vi "Main.vi"(11 "Module Admin":refnum<class "Delacor_lib_QMH_Module Admin.lvclass">) -> ()   [LabVIEW 2025, in "TS Environment Manager.lvlib"]
doc: "This template is based off of the Queued Message Handler design pattern and the Queued Message Handler project template that ships with LabVIEW.\n\nThe main difference is that the queue is private to this module and communication between modules is performed via Broadcast and Request events.\n\nRequest events are wrapped in public API methods and are handled in the Event Handling Loop (EHL) of this VI. Any module can register for Broadcast events sent by this module. The EHL generates messages based on user interface actions.\n\nThe Message Handling Loop (MHL) processes messages generated by the EHL, or by other messages. The messages are string values, so new messages can be added easily to the Message Cases case structure in the MHL. Each message cluster can also provide an optional value for Message Data, which is a variant that can be converted to whatever message-specific data is required.\n_____\nBased on DQMH Dev Tools: Project Template 7.1.1.1528."
uses:
  TS Environment Manager.lvlib
  <vilib>/Delacor/Delacor QMH/Libraries/Module Admin_class/Delacor_lib_QMH_Module Admin.lvclass
  Module Data--cluster.ctl
  <vilib>/Delacor/Delacor QMH/Libraries/Message Queue_class/Delacor_lib_QMH_Message Queue.lvclass/Delacor_lib_QMH_Message Queue.ctl
  Stop Argument--cluster.ctl
  <vilib>/Delacor/Delacor QMH/Libraries/Module Admin_class/Delacor_lib_QMH_Module Admin.lvclass/Delacor_lib_QMH_Module Admin.ctl
  Get Installations Argument--cluster.ctl
  ITSDiscovery/ITSDiscovery.lvclass
  Get Installations (Reply Payload)--cluster.ctl
  Type Definitions/TSInstall--cluster.ctl
  Type Definitions/Architecture--enum.ctl
  Get Profiles File Argument--cluster.ctl
  Launch Sequence Editor Argument--cluster.ctl
  IProcess Executor/IProcess Executor.lvclass
  Launch Sequence Editor (Reply Payload)--cluster.ctl
  Activate Version Argument--cluster.ctl
  Activate Version (Reply Payload)--cluster.ctl
  Add Profile Argument--cluster.ctl
  Type Definitions/Profile--cluster.ctl
  Add Profile (Reply Payload)--cluster.ctl
  Get Profile(s) Argument--cluster.ctl
  Get Profile(s) (Reply Payload)--cluster.ctl
  Delete Profile Argument--cluster.ctl
  Delete Profile (Reply Payload)--cluster.ctl
  Set Profiles File Argument--cluster.ctl
  Set Profiles File (Reply Payload)--cluster.ctl
  <vilib>/Utility/miscctls.llb/LVPointTypeDef.ctl
  <vilib>/Delacor/Delacor QMH/Libraries/Message Queue_class/Delacor_lib_QMH_Enqueue Message (Single).vi
  <vilib>/Delacor/Delacor QMH/Libraries/Module Admin_class/Delacor_lib_QMH_Get External Launch.vi
  <vilib>/Utility/config.llb/Read Key (Path).vi
  <vilib>/Utility/config.llb/Write Key (Path).vi
  <vilib>/Delacor/Delacor QMH/Libraries/Message Queue_class/Delacor_lib_QMH_Message Queue.lvclass
  <vilib>/Utility/config.llb/NI_LVConfig.lvlib
  <userlib>/_OpenG.lib/file/file.llb/openg_file.lvlib
panel:
  out "error out":errorcluster
  out "Status":string
  in  "Simulate MHL Error":bool
  in  "Simulate EHL Error":bool
  # "Other processes communicate with this Module via its Public API (wrappers for its Request Events).\n\nThis Module communicates with other processes via its Broadcast Events.\nAny process that wants to receive these messages can register for this module's Broadcast events."
  # "This template is for the DQMH framework. See the block diagram for more information on how to use this template."
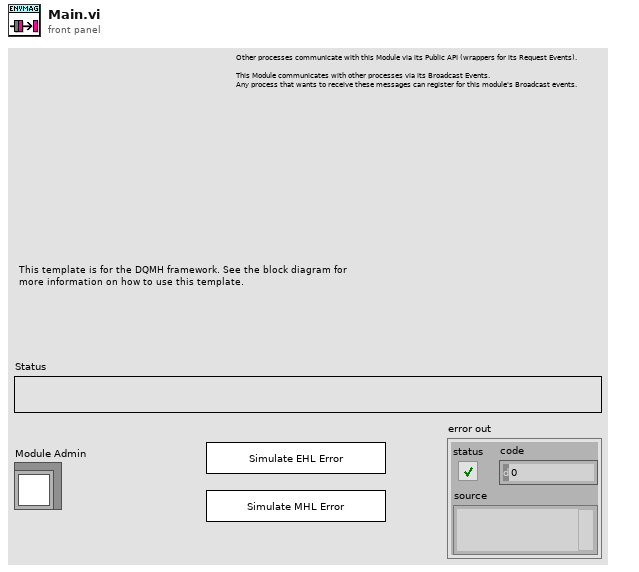
[diagram p1: front panel]
types:
  T1 = typedef "TS Environment Manager.lvlib/Request Events--cluster.ctl" = cluster{"Stop Module":refnum<user-event>, "Show Panel":refnum<user-event>, "Hide Panel":refnum<user-event>, "Get Module Execution Status":refnum<user-event>, "Show Diagram":refnum<user-event>, "Get Installations":refnum<user-event>, "Private.Get Profiles File":refnum<user-event>, "Launch Sequence Editor":refnum<user-event>, "Activate Version":refnum<user-event>, "Add Profile":refnum<user-event>, "Get Profile(s)":refnum<user-event>, "Delete Profile":refnum<user-event>, "Set Profiles File":refnum<user-event>}
  T2 = typedef "TS Environment Manager.lvlib/Module Data--cluster.ctl" = cluster{"Status":string, "Profile File":path}
  T3 = enum32{"invalid lock state", "Not Locked", "Locked (No Password)", "Password-protected"}
  T4 = typedef "TS Environment Manager.lvlib/Stop Argument--cluster.ctl" = cluster{"Origin":string, "Exit via Stop Module Req?":bool, "Wait for Module to stop?":bool}
  T5 = typedef "TS Environment Manager.lvlib/Get Installations Argument--cluster.ctl" = cluster{"ITSDiscovery.lvclass":refnum<class "ITSDiscovery.lvclass">, "Wait Notifier":refnum<notifier>, "wait for reply":bool}
  T6 = typedef "TS Environment Manager.lvlib/Get Profiles File Argument--cluster.ctl" = cluster{"Boolean":bool}
  T7 = typedef "TS Environment Manager.lvlib/Launch Sequence Editor Argument--cluster.ctl" = cluster{"ITSDiscovery.lvclass":refnum<class "ITSDiscovery.lvclass">, "IProcess Executor.lvclass":refnum<class "IProcess Executor.lvclass">, "Version":string, "Architecture":T8, "Environment":path, "Wait Notifier":refnum<notifier>, "wait for reply":bool}
  T8 = typedef "Architecture--enum.ctl" = enum16{"32bit", "64bit"}
  T9 = typedef "TS Environment Manager.lvlib/Activate Version Argument--cluster.ctl" = cluster{"Version":string, "IProcess Executor.lvclass":refnum<class "IProcess Executor.lvclass">, "ITSDiscovery.lvclass":refnum<class "ITSDiscovery.lvclass">, "Wait Notifier":refnum<notifier>, "wait for reply":bool}
  T10 = typedef "TS Environment Manager.lvlib/Add Profile Argument--cluster.ctl" = cluster{"Profile":T11, "Wait Notifier":refnum<notifier>, "wait for reply":bool}
  T11 = typedef "Profile--cluster.ctl" = cluster{"Name":string, "Version":string, "Architecture":T8, "Environment":path}
  T12 = typedef "TS Environment Manager.lvlib/Get Profile(s) Argument--cluster.ctl" = cluster{"Name":string, "Wait Notifier":refnum<notifier>, "wait for reply":bool}
  T13 = typedef "TS Environment Manager.lvlib/Delete Profile Argument--cluster.ctl" = cluster{"Name":string, "Wait Notifier":refnum<notifier>, "wait for reply":bool}
  T14 = typedef "TS Environment Manager.lvlib/Set Profiles File Argument--cluster.ctl" = cluster{"File Path":path, "Wait Notifier":refnum<notifier>, "wait for reply":bool}
  T15 = typedef "LVPointTypeDef.ctl" = cluster{"Horizontal":i16, "Vertical":i16}
  T16 = enum32{"Invalid", "Standard", "Closed", "Hidden", "Minimized", "Maximized"}
  T17 = typedef "TS Environment Manager.lvlib/Get Installations (Reply Payload)--cluster.ctl" = cluster{"Installations":T18[], "error":errorcluster}
  T18 = typedef "TSInstall--cluster.ctl" = cluster{"Version":string, "Architecture":T8, "Version Key":string, "ID":string}
  T19 = typedef "TS Environment Manager.lvlib/Get Profile(s) (Reply Payload)--cluster.ctl" = cluster{"Profile(s)":T11[], "File":path, "error":errorcluster}
  T20 = typedef "TS Environment Manager.lvlib/Add Profile (Reply Payload)--cluster.ctl" = cluster{"error":errorcluster}
  T21 = typedef "TS Environment Manager.lvlib/Activate Version (Reply Payload)--cluster.ctl" = cluster{"error":errorcluster, "Version":string}
  T22 = typedef "TS Environment Manager.lvlib/Launch Sequence Editor (Reply Payload)--cluster.ctl" = cluster{"error":errorcluster, "Version":string, "Architecture":T8, "Environment":path}
  T23 = typedef "TS Environment Manager.lvlib/Delete Profile (Reply Payload)--cluster.ctl" = cluster{"error":errorcluster}
  T24 = typedef "TS Environment Manager.lvlib/Set Profiles File (Reply Payload)--cluster.ctl" = cluster{"error":errorcluster}
  T25 = typedef "NI_LVConfig.lvlib/Config Data RefNum.ctl" = refnum<k1>
  T26 = typedef "Execution Plan--cluster.ctl" = cluster{"Exe Path":path, "Args":string[], "Timeout":i32}
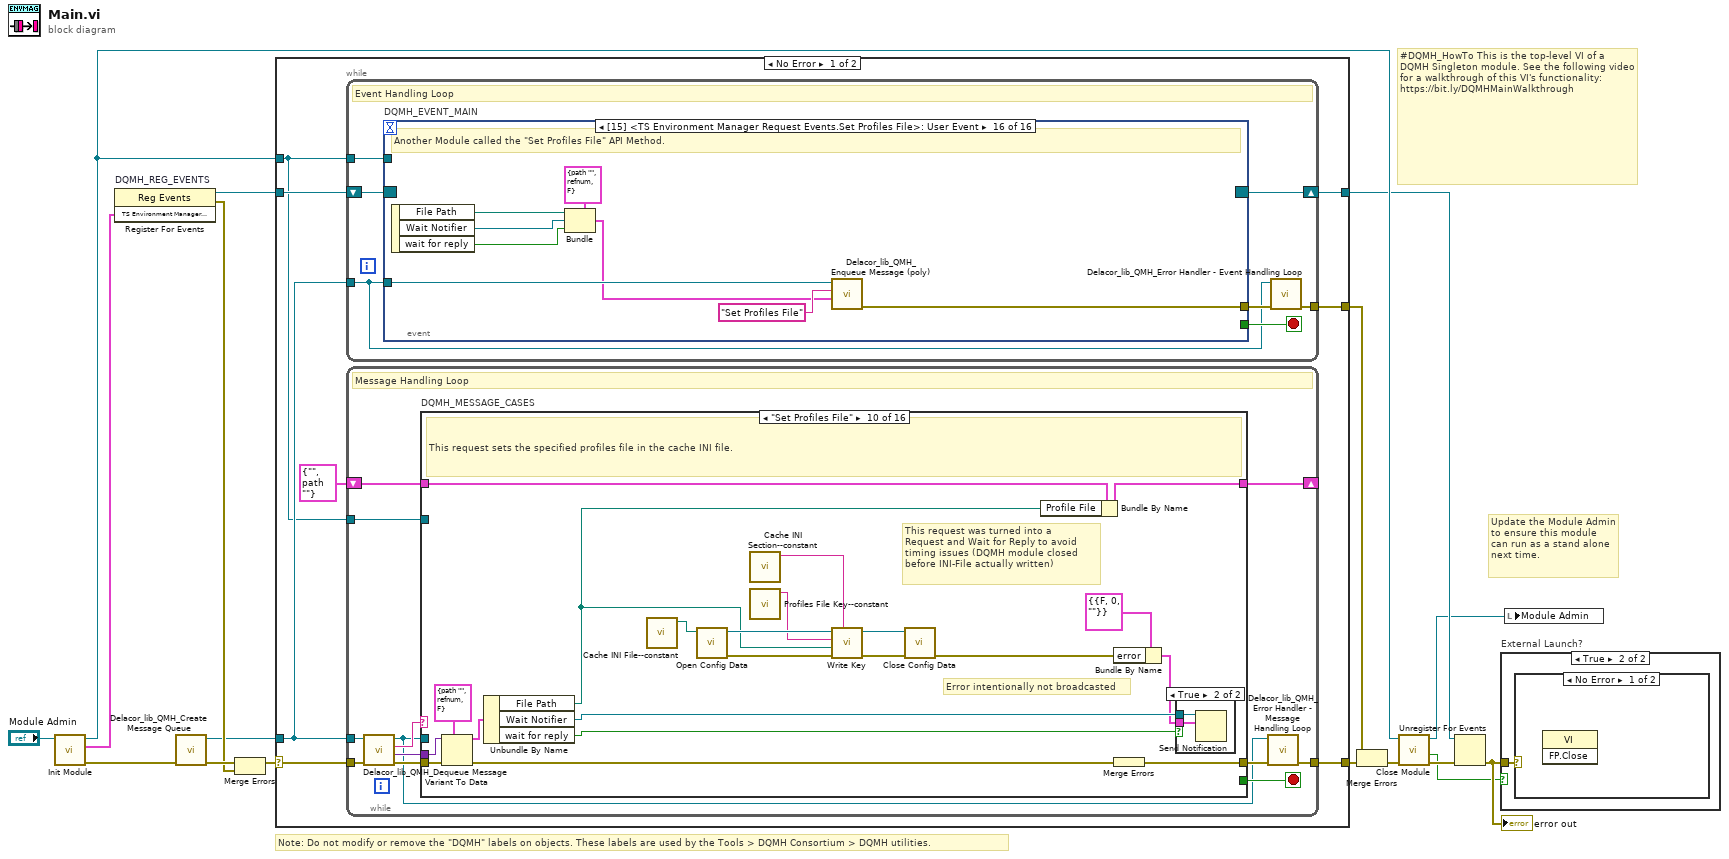
[diagram p0: block diagram]
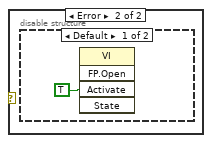
[diagram p3: hidden frame]
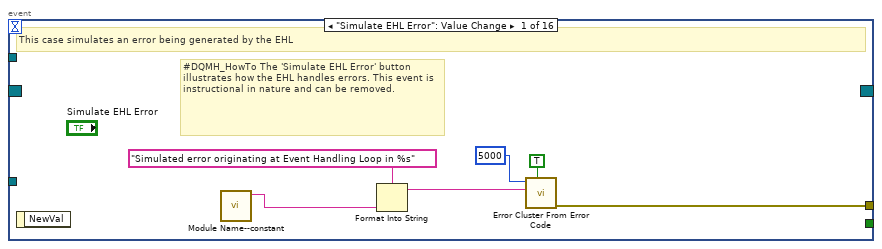
[diagram p5: hidden frame]
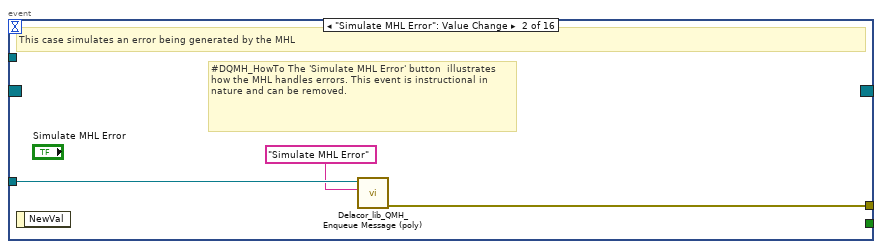
[diagram p6: hidden frame]
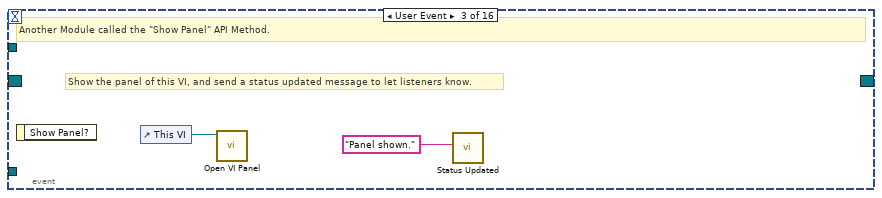
[diagram p7: hidden frame]
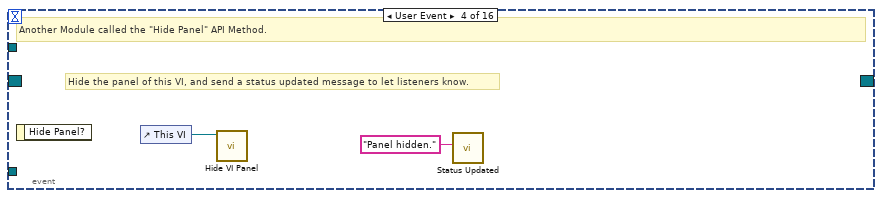
[diagram p8: hidden frame]
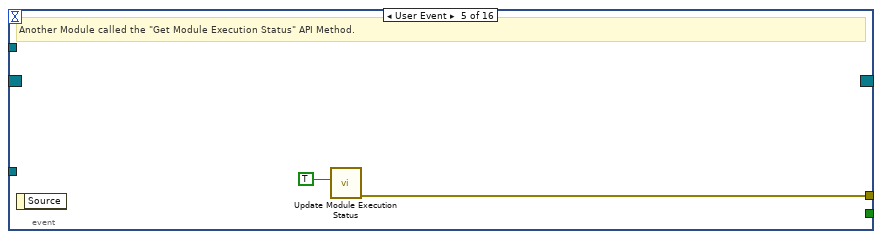
[diagram p9: hidden frame]
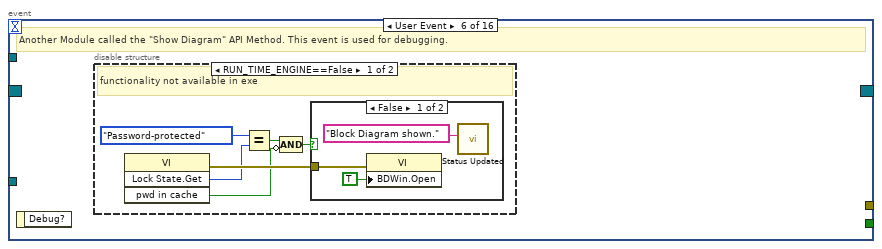
[diagram p10: hidden frame]
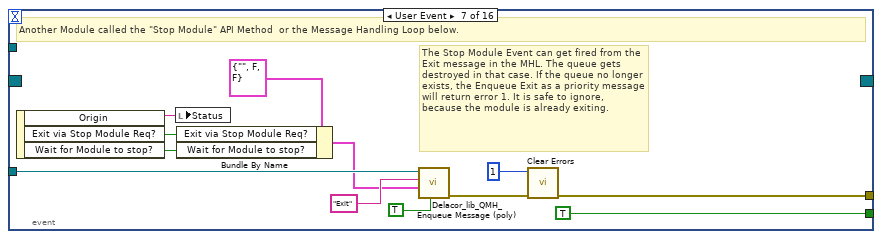
[diagram p13: hidden frame]
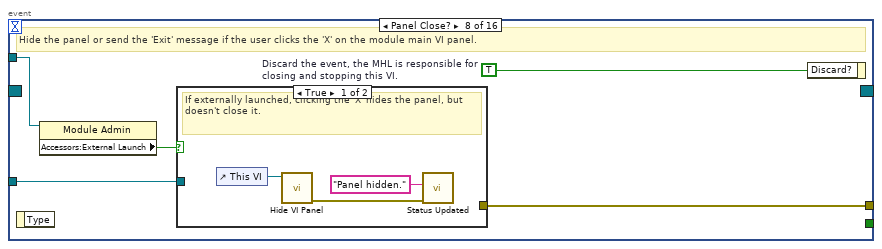
[diagram p14: hidden frame]
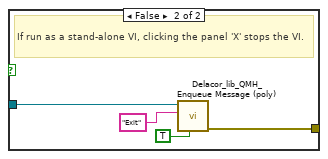
[diagram p15: hidden frame]
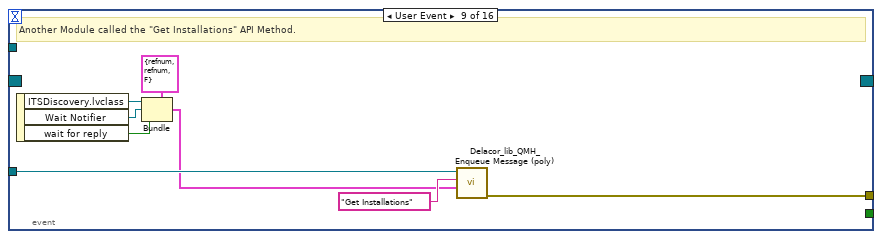
[diagram p16: hidden frame]
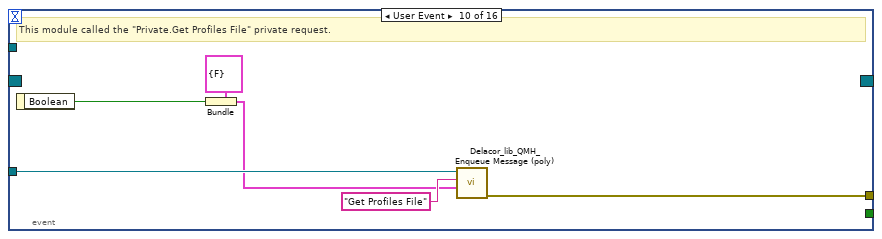
[diagram p17: hidden frame]
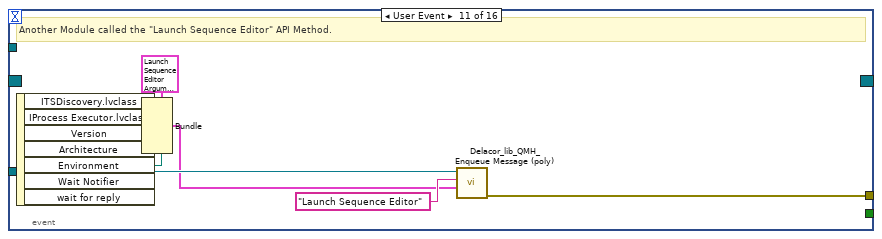
[diagram p18: hidden frame]
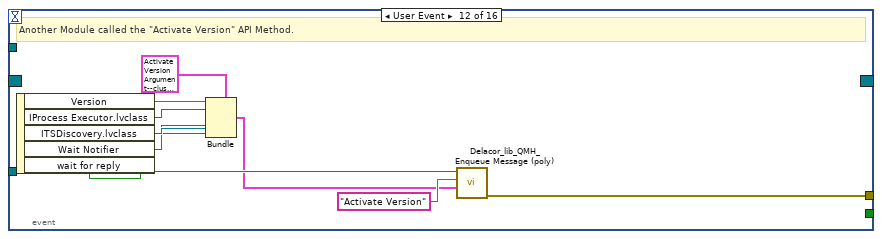
[diagram p19: hidden frame]
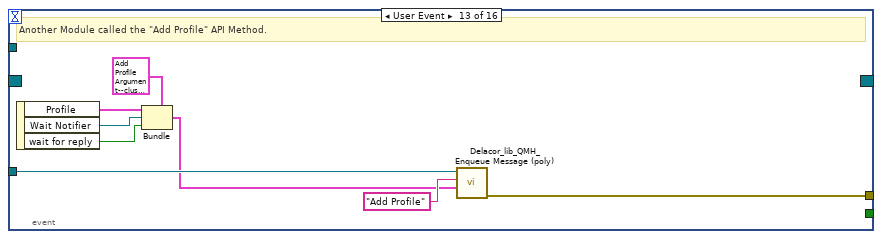
[diagram p20: hidden frame]
diagram:
  # "#DQMH_HowTo This is the top-level VI of a DQMH Singleton module. See the following video for a walkthrough of this VI's functionality: https://bit.ly/DQMHMainWalkthrough"
  # "Note: Do not modify or remove the \"DQMH\" labels on objects. These labels are used by the Tools > DQMH Consortium > DQMH utilities."
  # "Update the Module Admin to ensure this module can run as a stand alone next time."
  n1 = call "Init Module.vi"("Singleton Module Admin in"="Module Admin") -> ("error out"=w16:errorcluster, "TS Environment Manager Request Events"=w5:T1, "Singleton Module Admin out"=w8:refnum<class "Delacor_lib_QMH_Module Admin.lvclass">)  [unwired: 8 in]
  n2 = register-events "DQMH_REG_EVENTS"(w5) -> (reference out=w6:refnum<event-registration>, error out=w9:errorcluster)  [unwired: 2 in]
  n3 = call <vilib>:"Delacor_lib_QMH_Create Message Queue.vi"("error in"=w16) -> ("error out"=w11:errorcluster, "Message Queue"=w4:refnum<class "Delacor_lib_QMH_Message Queue.lvclass">)  [unwired: 9 in]
  n4 = Merge Errors(w11, w9) -> (w10:errorcluster)
  n5 = case shown="No Error" w10 {
    selector: w10 -> [w23 w438]
    tunnel: [w25 w437] -> w17
    tunnel: [w22 w436] -> w7
    tunnel: w6 -> [w20 w436]
    tunnel: w4 -> [w19 w431]
    tunnel: [w24 _] -> w14
    tunnel: w8 -> [w18 w432]
    frame No Error {
      n6 = while {
        tunnel: w19 -> [w26]
        shift-right: [w29] -> w22
        shift-left: w20 -> [w30]
        tunnel: [w31] -> w24
        tunnel: w18 -> [w27]
        stop <- w28 stop-if-true
        # "Event Handling Loop"
        n7 = event "DQMH_EVENT_MAIN" shown="[15] <TS Environment Manager Request Events.Set Profiles File>: User Event" {
          selector: w30 -> [_ _ _ _ _ _ _ _ _ _ _ _ _ _ _ _]
          dyn-events: [_ _ _ _ _ _ _ _ _ _ _ _ _ _ _ _] -> w29
          timeout: _ -> [_ _ _ _ _ _ _ _ _ _ _ _ _ _ _ _]
          tunnel: [_ _ _ _ _ _ TRUE ("Discard?") _ _ _ _ _ _ _ _ _] -> w28
          tunnel: w26 -> [_ w40 _ _ _ _ w64 w71 w88 w94 w106 w116 w124 w132 w140 w148]
          tunnel: [w38 w41 _ _ w47 _ w67 w73 w81 w89 w97 w109 w120 w125 w135 w143] -> w32
          tunnel: w27 -> [_ _ _ _ _ _ _ w70 _ _ _ _ _ _ _ _]
          event "Simulate EHL Error": Value Change {
            # "#DQMH_HowTo The 'Simulate EHL Error' button  illustrates how the EHL handles errors. This event is instructional in nature and can be removed."
            # "This case simulates an error being generated by the EHL"
            n8 = event-data() -> ()  [unwired: 1 in, 1 out]
            n9 = call "Module Name--constant.vi"() -> ("Module Name"=w35:string)  [unwired: 11 in]
            n10 = Format Into String(format string="Simulated error originating at Event Handling Loop in %s", w35) -> (resulting string=w36:string)  [unwired: 2 in, 1 out]
            n11 = call <vilib>:"Error Cluster From Error Code.vi"("show call chain? (False)"=TRUE, "error message (\"\")"=w36, "error code (0)"=5000) -> ("error out"=w38:errorcluster)  [unwired: 6 in]
          }
          event "Simulate MHL Error": Value Change {
            # "#DQMH_HowTo The 'Simulate MHL Error' button  illustrates how the MHL handles errors. This event is instructional in nature and can be removed."
            # "This case simulates an error being generated by the MHL"
            n12 = event-data() -> ()  [unwired: 1 in, 1 out]
            n13 = call-poly <vilib>:"Delacor_lib_QMH_Enqueue Message (poly).vi"("Message"="Simulate MHL Error", "Message Queue in"=w40) -> ("error out"=w41:errorcluster)  [unwired: 8 in, 1 out]
          }
          event User Event {
            # "Show the panel of this VI, and send a status updated message to let listeners know."
            # "Another Module called the \"Show Panel\" API Method."
            n14 = event-data() -> ()  [unwired: 1 in, 1 out]
            n15 = control-ref of="This VI"() -> (w43:refnum<vi>)
            n16 = call "Open VI Panel.vi"("VI"=w43) -> ()  [unwired: 10 in, 1 out]
            n17 = call "Status Updated.vi"("Status"="Panel shown." ("format string")) -> ()  [unwired: 10 in, 1 out]
          }
          event User Event {
            # "Hide the panel of this VI, and send a status updated message to let listeners know."
            # "Another Module called the \"Hide Panel\" API Method."
            n18 = event-data() -> ()  [unwired: 1 in, 1 out]
            n19 = control-ref of="This VI"() -> (w45:refnum<vi>)
            n20 = call "Hide VI Panel.vi"("VI"=w45) -> ()  [unwired: 10 in, 1 out]
            n21 = call "Status Updated.vi"("Status"="Panel hidden." ("format string")) -> ()  [unwired: 10 in, 1 out]
          }
          event User Event {
            # "Another Module called the \"Get Module Execution Status\" API Method."
            n22 = event-data() -> ()  [unwired: 1 in, 1 out]
            n23 = call "Update Module Execution Status.vi"("Running?"=TRUE) -> ("error out"=w47:errorcluster)  [unwired: 10 in]
          }
          event User Event {
            # "Another Module called the \"Show Diagram\" API Method. This event is used for debugging."
            n24 = event-data() -> ()  [unwired: 1 in, 1 out]
            n25 = disable-structure shown="RUN_TIME_ENGINE==False" {
              frame condition #0 (active) {
                # "functionality not available in exe"
                n26 = invoke on="Invoke Node" class="VI" method="Lock State.Get"() -> (error out=w53:errorcluster, "Get Lock State"=w52:T3, "pwd in cache"=w49:bool)  [unwired: 4 in, 1 out]
                n27 = Equal?(x=T3."Password-protected", y=w52) -> (x = y?=w50:bool)
                n28 = Compound Arithmetic op=AND(w50, invert w49) -> (w48:bool)
                n29 = case shown="False" w48 {
                  tunnel: w53 -> [w56 _]
                  frame False {
                    n30 = property on="Property Node" class="VI"(error in=w56, "BDWin.Open"=TRUE ("Block Diagram Window:Open")) -> ()  [unwired: 1 in, 2 out]
                    n31 = call "Status Updated.vi"("Status"="Block Diagram shown." ("format string")) -> ()  [unwired: 10 in, 1 out]
                  }
                  frame True {
                    # "Password-protected VI, and the password is not in the cache. Do not show the diagram."
                  }
                }
              }
              frame condition #1 {
              }
            }
          }
          event User Event {
            # "The Stop Module Event can get fired from the Exit message in the MHL. The queue gets destroyed in that case. If the queue no longer exists, the Enqueue Exit as a priority message will return error 1. It is safe to ignore, because the module is already exiting."
            # "Another Module called the \"Stop Module\" API Method  or the Message Handling Loop below."
            n32 = event-data() -> ("Origin"=w63:string, "Exit via Stop Module Req?"=w59:bool, "Wait for Module to stop?"=w58:bool)  [unwired: 1 in]
            n33 = local write "Status"(w63) -> ()
            n34 = Bundle By Name(cluster=T4 {"Origin"="", "Exit via Stop Module Req?"=FALSE, "Wait for Module to stop?"=FALSE} ("Stop Argument"), "Exit via Stop Module Req?"=w59, "Wait for Module to stop?"=w58) -> (w57:T4)
            n35 = call-poly <vilib>:"Delacor_lib_QMH_Enqueue Message (poly).vi"("Priority Message? (F)"=TRUE, "Message Data"=w57, "Message"="Exit", "Message Queue in"=w64) -> ("error out"=w68:errorcluster)  [unwired: 6 in, 1 out]
            n36 = call <vilib>:"Clear Errors.vi"("error in (no error)"=w68, "specific error code to clear (0: all)"=1) -> ("error out"=w67:errorcluster)  [unwired: 4 in, 1 out]
          }
          event Panel Close? {
            w72 = TRUE  # Discard the event, the MHL is responsible for closing and stopping this VI.
            # "Hide the panel or send the 'Exit' message if the user clicks the 'X' on the module main VI panel."
            n37 = event-data() -> ()  [unwired: 1 in, 1 out]
            n38 = property on="Property Node" class="Module Admin"(reference=w70) -> ("Accessors:External Launch"=w69:bool)  [unwired: 1 in, 2 out]
            n39 = case shown="True" w69 {
              tunnel: w71 -> [_ w79]
              tunnel: [_ w80] -> w73
              frame True {
                # "If externally launched, clicking the 'X' hides the panel, but doesn't close it."
                n40 = control-ref of="This VI"() -> (w76:refnum<vi>)
                n41 = call "Hide VI Panel.vi"("VI"=w76) -> ("error out"=w74:errorcluster)  [unwired: 10 in]
                n42 = call "Status Updated.vi"("error in"=w74, "Status"="Panel hidden." ("format string")) -> ()  [unwired: 9 in, 1 out]
              }
              frame False {
                # "If run as a stand-alone VI, clicking the panel 'X' stops the VI."
                n43 = call-poly <vilib>:"Delacor_lib_QMH_Enqueue Message (poly).vi"("Priority Message? (F)"=TRUE, "Message"="Exit", "Message Queue in"=w79) -> ("error out"=w80:errorcluster)  [unwired: 7 in, 1 out]
              }
            }
            n44 = event-data ("Event Filter Node")("Discard?"=w72) -> ()  [unwired: 1 in, 1 out]
          }
          event User Event {
            # "Another Module called the \"Get Installations\" API Method."
            n45 = event-data() -> ("ITSDiscovery.lvclass"=w84:refnum<class "ITSDiscovery.lvclass">, "Wait Notifier"=w83:refnum<notifier>, "wait for reply"=w82:bool)  [unwired: 1 in]
            n46 = Bundle(cluster=T5 {"ITSDiscovery.lvclass"=refnum, "Wait Notifier"=refnum, "wait for reply"=FALSE} ("Get Installations Argument"), "ITSDiscovery.lvclass"=w84, "Wait Notifier"=w83, "wait for reply"=w82) -> (w85:T5)
            n47 = call-poly <vilib>:"Delacor_lib_QMH_Enqueue Message (poly).vi"("Message Data"=w85, "Message"="Get Installations", "Message Queue in"=w88) -> ("error out"=w81:errorcluster)  [unwired: 7 in, 1 out]
          }
          event User Event {
            # "This module called the \"Private.Get Profiles File\" private request."
            n48 = event-data() -> ("Boolean"=w90:bool)  [unwired: 1 in]
            n49 = Bundle(cluster=T6 {"Boolean"=FALSE} ("Get Profile Argument"), "Boolean"=w90) -> (w91:T6)
            n50 = call-poly <vilib>:"Delacor_lib_QMH_Enqueue Message (poly).vi"("Message Data"=w91, "Message"="Get Profiles File", "Message Queue in"=w94) -> ("error out"=w89:errorcluster)  [unwired: 7 in, 1 out]
          }
          event User Event {
            # "Another Module called the \"Launch Sequence Editor\" API Method."
            n51 = event-data() -> ("ITSDiscovery.lvclass"=w102:refnum<class "ITSDiscovery.lvclass">, "IProcess Executor.lvclass"=w101:refnum<class "IProcess Executor.lvclass">, "Version"=w100:string, "Architecture"=w99:T8, "Environment"=w98:path, "Wait Notifier"=w96:refnum<notifier>, "wait for reply"=w95:bool)  [unwired: 1 in]
            n52 = Bundle(cluster=T7 {"ITSDiscovery.lvclass"=refnum, "IProcess Executor.lvclass"=refnum, "Version"="", "Architecture"=enum."32bit", "Environment"=path "", "Wait Notifier"=refnum, "wait for reply"=FALSE} ("Launch Sequence Editor Argument"), "ITSDiscovery.lvclass"=w102, "IProcess Executor.lvclass"=w101, "Version"=w100, "Architecture"=w99, "Environment"=w98, "Wait Notifier"=w96, "wait for reply"=w95) -> (w103:T7)
            n53 = call-poly <vilib>:"Delacor_lib_QMH_Enqueue Message (poly).vi"("Message Data"=w103, "Message"="Launch Sequence Editor", "Message Queue in"=w106) -> ("error out"=w97:errorcluster)  [unwired: 7 in, 1 out]
          }
          event User Event {
            # "Another Module called the \"Activate Version\" API Method."
            n54 = event-data() -> ("Version"=w112:string, "IProcess Executor.lvclass"=w111:refnum<class "IProcess Executor.lvclass">, "ITSDiscovery.lvclass"=w110:refnum<class "ITSDiscovery.lvclass">, "Wait Notifier"=w108:refnum<notifier>, "wait for reply"=w107:bool)  [unwired: 1 in]
            n55 = Bundle(cluster=T9 {"Version"="", "IProcess Executor.lvclass"=refnum, "ITSDiscovery.lvclass"=refnum, "Wait Notifier"=refnum, "wait for reply"=FALSE} ("Activate Version Argument"), "Version"=w112, "IProcess Executor.lvclass"=w111, "ITSDiscovery.lvclass"=w110, "Wait Notifier"=w108, "wait for reply"=w107) -> (w113:T9)
            n56 = call-poly <vilib>:"Delacor_lib_QMH_Enqueue Message (poly).vi"("Message Data"=w113, "Message"="Activate Version", "Message Queue in"=w116) -> ("error out"=w109:errorcluster)  [unwired: 7 in, 1 out]
          }
          event User Event {
            # "Another Module called the \"Add Profile\" API Method."
            n57 = event-data() -> ("Profile"=w119:T11, "Wait Notifier"=w118:refnum<notifier>, "wait for reply"=w117:bool)  [unwired: 1 in]
            n58 = Bundle(cluster=T10 {"Profile"={"Name"="", "Version"="", "Architecture"=enum."32bit", "Environment"=path ""}, "Wait Notifier"=refnum, "wait for reply"=FALSE} ("Add Profile Argument"), "Profile"=w119, "Wait Notifier"=w118, "wait for reply"=w117) -> (w121:T10)
            n59 = call-poly <vilib>:"Delacor_lib_QMH_Enqueue Message (poly).vi"("Message Data"=w121, "Message"="Add Profile", "Message Queue in"=w124) -> ("error out"=w120:errorcluster)  [unwired: 7 in, 1 out]
          }
          event User Event {
            # "Another Module called the \"Get Profile(s)\" API Method."
            n60 = event-data() -> ("Name"=w128:string, "Wait Notifier"=w127:refnum<notifier>, "wait for reply"=w126:bool)  [unwired: 1 in]
            n61 = Bundle(cluster=T12 {"Name"="", "Wait Notifier"=refnum, "wait for reply"=FALSE} ("Get Profile(s) Argument"), "Name"=w128, "Wait Notifier"=w127, "wait for reply"=w126) -> (w129:T12)
            n62 = call-poly <vilib>:"Delacor_lib_QMH_Enqueue Message (poly).vi"("Message Data"=w129, "Message"="Get Profile(s)", "Message Queue in"=w132) -> ("error out"=w125:errorcluster)  [unwired: 7 in, 1 out]
          }
          event User Event {
            # "Another Module called the \"Delete Profile\" API Method."
            n63 = event-data() -> ("Name"=w136:string, "Wait Notifier"=w134:refnum<notifier>, "wait for reply"=w133:bool)  [unwired: 1 in]
            n64 = Bundle(cluster=T13 {"Name"="", "Wait Notifier"=refnum, "wait for reply"=FALSE} ("Delete Profile Argument"), "Name"=w136, "Wait Notifier"=w134, "wait for reply"=w133) -> (w137:T13)
            n65 = call-poly <vilib>:"Delacor_lib_QMH_Enqueue Message (poly).vi"("Message Data"=w137, "Message"="Delete Profile", "Message Queue in"=w140) -> ("error out"=w135:errorcluster)  [unwired: 7 in, 1 out]
          }
          event User Event {
            # "Another Module called the \"Set Profiles File\" API Method."
            n66 = event-data() -> ("File Path"=w144:path, "Wait Notifier"=w142:refnum<notifier>, "wait for reply"=w141:bool)  [unwired: 1 in]
            n67 = Bundle(cluster=T14 {"File Path"=path "", "Wait Notifier"=refnum, "wait for reply"=FALSE} ("Set Profiles File Argument"), "File Path"=w144, "Wait Notifier"=w142, "wait for reply"=w141) -> (w145:T14)
            n68 = call-poly <vilib>:"Delacor_lib_QMH_Enqueue Message (poly).vi"("Message Data"=w145, "Message"="Set Profiles File", "Message Queue in"=w148) -> ("error out"=w143:errorcluster)  [unwired: 7 in, 1 out]
          }
        }
        n69 = call-dynamic "Delacor_lib_QMH_Error Handler - Event Handling Loop.vi"("error in"=w32, "Message Queue in"=w26) -> ("dup error in"=w31:errorcluster)  [unwired: 8 in, 1 out]
      }
      n70 = while {
        tunnel: w19 -> [w149]
        shift-right: [w157] -> _
        shift-left: T2 {"Status"="", "Profile File"=path ""} ("Data Cluster") -> [w158]
        tunnel: w23 -> [w160]
        tunnel: [w152] -> w25
        tunnel: w18 -> [w153]
        stop <- w156 stop-if-true
        # "Message Handling Loop"
        n71 = call-dynamic "Delacor_lib_QMH_Dequeue Message.vi"("error in"=w160, "Message Queue in"=w149) -> ("error out"=w159:errorcluster, "Message Data"=w154:variant, "Message"=w155:string, "Message Queue out"=w150:refnum<class "Delacor_lib_QMH_Message Queue.lvclass">)  [unwired: 6 in]
        n72 = case "DQMH_MESSAGE_CASES" shown="\"Set Profiles File\"" w155 {
          selector: w155 -> [_ _ _ _ _ _ _ _ _ _ _ _ _ _ _ w426]
          tunnel: w150 -> [_ _ _ _ _ _ _ _ _ _ _ _ _ w392 w414 _]
          tunnel: w159 -> [w179 w183 w197 w220 w252 w289 w310 w333 w349 w372 w377 w379 w388 w399 w420 w429]
          tunnel: [w161 w183 w187 w210 w243 w280 w300 w323 w340 w363 w376 w379 w387 w395 w415 w430] -> w151
          tunnel: w158 -> [w170 w182 w196 w216 w242 w278 w309 w332 w339 w354 w375 w378 w385 w394 w413 w427]
          tunnel: [w169 w182 w196 w217 w242 w278 w309 w332 w339 w355 w375 w378 w385 w394 w413 w427] -> w157
          tunnel: [_ _ _ _ _ _ _ _ _ _ _ _ _ _ w412 _] -> w156
          tunnel: w154 -> [_ _ w194 w219 w250 w287 w307 w330 w347 w370 _ _ _ w393 w411 _]
          tunnel: w153 -> [w171 _ _ _ _ _ _ _ _ _ _ _ _ w391 w406 _]
          frame "Initialize" {
            w165 = "Initial Message" ("Initial Message")
            # "#DQMH_CodeNeeded - Initialize the appearance of the front panel."
            # "#DQMH_CodeNeeded - Initialize your state data here."
            # "Initialize - Any operation that needs to be done before the module can receive messages. Synchronize Caller Events.vi will inform Start Module.vi that the module has launched and is ready to receive messages. Module Did Init.vi will broadcast that the module initialized."
            n73 = call "Synchronize Caller Events.vi"("error in"=w179, "Singleton Module Admin in"=w171) -> ("error out"=w163:errorcluster, "Singleton Module Admin out"=w166:refnum<class "Delacor_lib_QMH_Module Admin.lvclass">)  [unwired: 8 in]
            n74 = property on="Property Node" class="Module Admin"(reference=w166) -> ("Accessors:External Launch"=w175:bool)  [unwired: 1 in, 2 out]
            n75 = Select(t=T16."Hidden" ("State"), s=w175, f=T16."Standard" ("State")) -> (s? t:f=w172:T16)
            n76 = call "Module Name--constant.vi"() -> ("Module Name"=w178:string)  [unwired: 11 in]
            n77 = property on="Property Node" class="VI"("Front Panel.Title"=w178) -> (reference out=w177:refnum<vi>, error out=w181:errorcluster)  [unwired: 2 in]
            n78 = invoke on="Invoke Node" class="VI" method="FP.Open"(reference=w177, error in=w181, "State"=w172) -> (reference out=w176:refnum<vi>, error out=w180:errorcluster)  [unwired: 2 in, 3 out]
            n79 = Bundle By Name(cluster=w170, "Status"=w165) -> (w169:T2)
            n80 = invoke on="Invoke Node" class="VI" method="FP.Center"(reference=w176, error in=w180) -> ()  [unwired: 1 in, 3 out]
            n81 = property on="Pane" class="Pane"("Origin"=T15 {"Horizontal"=0, "Vertical"=0}) -> ()  [unwired: 2 in, 2 out]
            n82 = call "Module Name--constant.vi"() -> ("Module Name"=w167:string)  [unwired: 11 in]
            n83 = call "Module Did Init.vi"("error in"=w163, "Initialized?"=TRUE, "Origin"=w167) -> ("error out"=w162:errorcluster)  [unwired: 8 in]
            n84 = call "Get Profiles File.vi"("error in"=w162) -> ("error out"=w161:errorcluster)  [unwired: 10 in]
            "Status" <- w165
          }
          frame "---Module Specific---" {
            # "Separator -- The following cases handle messages specific to this Module."
          }
          frame "Get Installations" {
            # "This event retrieves all TestStand Installations in the systems and returns them as an array of TSInstall elements."
            n85 = Variant To Data(error in=w197, type=T5 {"ITSDiscovery.lvclass"=refnum, "Wait Notifier"=refnum, "wait for reply"=FALSE} ("Get Installations Argument"), Variant=w194) -> (data=w192:T5, error out=w195:errorcluster)
            n86 = Unbundle By Name(w192) -> ("ITSDiscovery.lvclass"=w186:refnum<class "ITSDiscovery.lvclass">, "Wait Notifier"=w191:refnum<notifier>, "wait for reply"=w190:bool)
            n87 = call-dynamic "Find Installs.vi"("ITSDiscovery in"=w186) -> ("error out"=w184:errorcluster, "TSInstalls Out"=w185:T18[])  [unwired: 9 in]
            n88 = Bundle By Name(cluster=T17 {"Installations"=[], "error"={"status"=FALSE, "code"=0, "source"=""}} ("Get Installations (Reply Payload)"), "Installations"=w185, "error"=w184) -> (w189:T17)
            n89 = Merge Errors(w195) -> (w187:errorcluster)
            n90 = case "DQMH_FIRE_NOTIFIER" shown="True" w190 {
              tunnel: w191 -> [_ w199]
              tunnel: w189 -> [_ w198]
              frame False {
              }
              frame True {
                n91 = Send Notification(notification=w198, notifier=w199) -> ()  [unwired: 1 in, 2 out]
              }
            }
          }
          frame "Get Profiles File" {
            # "This event reads the configured profile file location from the cache file.\nIf the entry is not found, it is created with the default value <i>C:\\Users\\<user>\\Environment Toolkit Profiles.ini</i>."
            n92 = Variant To Data(error in=w220, type=T6 {"Boolean"=FALSE} ("Get Profile Argument"), Variant=w219) -> (error out=w215:errorcluster)  [unwired: 1 out]
            n93 = call "Cache INI File--constant.vi"() -> ("Cache INI File"=w214:path)  [unwired: 11 in]
            n94 = call <vilib>:"Open Config Data.vi"("error in (no error)"=w215, "create file if necessary (T)"=TRUE, "configuration file path"=w214) -> ("error out"=w212:errorcluster, "refnum"=w211:T25)  [unwired: 6 in, 1 out]
            n95 = call "Cache INI Section--constant.vi"() -> ("Cache INI Section"=w205:string)  [unwired: 11 in]
            n96 = call "Profiles File Key--constant.vi"() -> ("Profiles File Key"=w204:string)  [unwired: 11 in]
            n97 = call-poly <vilib>:"Read Key.vi"("section"=w205, "error in (no error)"=w212, "default value"=path "", "key"=w204, "refnum"=w211) -> ("error out"=w208:errorcluster, "value"=w200:path, "refnum out"=w206:T25)  [unwired: 3 in, 1 out]
            n98 = Empty String/Path?(string/path=w200) -> (empty?=w207:bool)
            n99 = case shown="False" w207 {
              tunnel: w208 -> [w221 w230]
              tunnel: w206 -> [w222 w229]
              tunnel: w205 -> [_ w228]
              tunnel: w204 -> [_ w227]
              tunnel: [w222 w226] -> w203
              tunnel: [w221 w225] -> w202
              tunnel: [w223 w224] -> w201
              tunnel: w200 -> [w223 _]
              frame False {
                # "Entry found, use value"
              }
              frame True {
                # "No entry --> Create with standard value"
                n100 = call "Default Profiles File Path--constant.vi"() -> ("Default Profiles File Path"=w224:path)  [unwired: 11 in]
                n101 = call-poly <vilib>:"Write Key.vi"("section"=w228, "error in (no error)"=w230, "value"=w224, "key"=w227, "refnum"=w229) -> ("error out"=w225:errorcluster, "refnum out"=w226:T25)  [unwired: 4 in, 1 out]
              }
            }
            n102 = Bundle By Name(cluster=w216, "Profile File"=w201) -> (w217:T2)
            n103 = call <vilib>:"Close Config Data.vi"("error in (no error)"=w202, "refnum"=w203) -> ("error out"=w210:errorcluster)  [unwired: 8 in, 1 out]
          }
          frame "Get Profile(s)" {
            # "This event allows the user to retrieve the current profile file followed by the specified profile (if specified) or all profiles if no name is specified."
            n104 = Variant To Data(error in=w252, type=T12 {"Name"="", "Wait Notifier"=refnum, "wait for reply"=FALSE} ("Get Profile(s) Argument"), Variant=w250) -> (data=w248:T12, error out=w251:errorcluster)
            n105 = Unbundle By Name(w242) -> ("Profile File"=w233:path)
            n106 = Unbundle By Name(w248) -> ("Name"=w239:string, "Wait Notifier"=w247:refnum<notifier>, "wait for reply"=w246:bool)
            n107 = Strip Path(path=w233) -> (stripped path=w232:path)  [unwired: 1 out]
            n108 = call <userlib>:"Create Dir if Non-Existant__ogtk.vi"("Directory Path"=w232) -> ("error out"=w231:errorcluster)  [unwired: 8 in, 2 out]
            n109 = call <vilib>:"Open Config Data.vi"("error in (no error)"=w231, "configuration file path"=w233) -> ("error out"=w236:errorcluster, "refnum"=w237:T25)  [unwired: 7 in, 1 out]
            n110 = Empty String/Path?(string/path=w239) -> (empty?=w238:bool)
            n111 = case shown="True" w238 {
              tunnel: w237 -> [w259 w267]
              tunnel: w236 -> [w257 w266]
              tunnel: [w253 w262] -> w241
              tunnel: [w256 w261] -> w235
              tunnel: [w255 w260] -> w234
              tunnel: w239 -> [w258 _]
              frame False {
                # "Read only specified profile"
                n112 = call "Read Profile.vi"("error in"=w257, "Name"=w258, "File in"=w259) -> ("error out"=w255:errorcluster, "Profile"=w254:T11, "File out"=w256:T25)  [unwired: 6 in]
                n113 = Build Array(w254) -> (w253:T11[])
              }
              frame True {
                # "User did not specify name: read all profiles"
                n114 = call <vilib>:"Get Section Names.vi"("error in (no error)"=w266, "refnum"=w267) -> ("error out"=w264:errorcluster, "section names"=w263:string[], "refnum out"=w265:T25)  [unwired: 7 in]
                n115 = for {
                  shift-right: [w270] -> w260
                  shift-left: w264 -> [w271]
                  tunnel: w263 -> [w272] mode=indexing
                  tunnel: [w269] -> w262 mode=indexing
                  shift-right: [w268] -> w261
                  shift-left: w265 -> [w273]
                  # "Iterate through sections (names) and read profiles"
                  n116 = call "Read Profile.vi"("error in"=w271, "Name"=w272, "File in"=w273) -> ("error out"=w270:errorcluster, "Profile"=w269:T11, "File out"=w268:T25)  [unwired: 6 in]
                }
              }
            }
            n117 = call <vilib>:"Close Config Data.vi"("error in (no error)"=w234, "refnum"=w235) -> ("error out"=w240:errorcluster)  [unwired: 8 in, 1 out]
            n118 = Bundle By Name(cluster=T19 {"Profile(s)"=[], "File"=path "", "error"={"status"=FALSE, "code"=0, "source"=""}} ("Get Profile(s) (Reply Payload)"), "File"=w233, "Profile(s)"=w241, "error"=w240) -> (w245:T19)
            n119 = Merge Errors(w251) -> (w243:errorcluster)
            n120 = case "DQMH_FIRE_NOTIFIER" shown="True" w246 {
              tunnel: w247 -> [_ w275]
              tunnel: w245 -> [_ w274]
              frame False {
              }
              frame True {
                n121 = Send Notification(notification=w274, notifier=w275) -> ()  [unwired: 1 in, 2 out]
              }
            }
          }
          frame "Add Profile" {
            # "Error intentionally not propagated\nthrough error reported event"
            # "This request adds a profile to the active profile file."
            n122 = Variant To Data(error in=w289, type=T10 {"Profile"={"Name"="", "Version"="", "Architecture"=enum."32bit", "Environment"=path ""}, "Wait Notifier"=refnum, "wait for reply"=FALSE} ("Add Profile Argument"), Variant=w287) -> (data=w285:T10, error out=w288:errorcluster)
            n123 = Unbundle By Name(w285) -> ("Profile"=w277:T11, "Wait Notifier"=w284:refnum<notifier>, "wait for reply"=w283:bool)
            n124 = Unbundle By Name(w278) -> ("Profile File"=w279:path)
            n125 = call "Add Profile to File.vi"("Profile"=w277, "File Path"=w279) -> ("error out"=w276:errorcluster)  [unwired: 9 in]
            n126 = Bundle By Name(cluster=T20 {"error"={"status"=FALSE, "code"=0, "source"=""}} ("Add Profile (Reply Payload)"), "error"=w276) -> (w282:T20)
            n127 = Merge Errors(w288) -> (w280:errorcluster)
            n128 = case "DQMH_FIRE_NOTIFIER" shown="True" w283 {
              tunnel: w284 -> [_ w291]
              tunnel: w282 -> [_ w290]
              frame False {
              }
              frame True {
                n129 = Send Notification(notification=w290, notifier=w291) -> ()  [unwired: 1 in, 2 out]
              }
            }
          }
          frame "Activate Version" {
            # "Error input wired so that\nno broadcast is sent when\nan error occurrs"
            # "This event activates the specified TestStand version."
            n130 = Variant To Data(error in=w310, type=T9 {"Version"="", "IProcess Executor.lvclass"=refnum, "ITSDiscovery.lvclass"=refnum, "Wait Notifier"=refnum, "wait for reply"=FALSE} ("Activate Version Argument"), Variant=w307) -> (data=w305:T9, error out=w308:errorcluster)
            n131 = Unbundle By Name(w305) -> ("IProcess Executor.lvclass"=w294:refnum<class "IProcess Executor.lvclass">, "ITSDiscovery.lvclass"=w297:refnum<class "ITSDiscovery.lvclass">, "Version"=w293:string, "Wait Notifier"=w304:refnum<notifier>, "wait for reply"=w303:bool)
            n132 = call "Get TSInstall by Version (all architectures).vi"("Version"=w293, "ITSDiscovery in"=w297) -> ("error out"=w298:errorcluster, "TSInstall Out"=w296:T18)  [unwired: 8 in]
            n133 = call "Build TS Activation Execution Plan.vi"("error in"=w298, "TSInstall"=w296) -> ("error out"=w299:errorcluster, "Execution Plan"=w295:T26)  [unwired: 8 in]
            n134 = call-dynamic "Run.vi"("error in"=w299, "Execution Plan"=w295, "IProcess Executor in"=w294) -> ("error out"=w292:errorcluster)  [unwired: 7 in, 1 out]
            n135 = Bundle By Name(cluster=T21 {"error"={"status"=FALSE, "code"=0, "source"=""}, "Version"=""} ("Activate Version (Reply Payload)"), "Version"=w293, "error"=w292) -> (w302:T21)
            n136 = Merge Errors(w308, w292) -> (w300:errorcluster)
            n137 = call "Version Activated.vi"("error in"=w292, "Reply Payload"=w302) -> ()  [unwired: 9 in, 1 out]
            n138 = case "DQMH_FIRE_NOTIFIER" shown="True" w303 {
              tunnel: w304 -> [_ w312]
              tunnel: w302 -> [_ w311]
              frame False {
              }
              frame True {
                n139 = Send Notification(notification=w311, notifier=w312) -> ()  [unwired: 1 in, 2 out]
              }
            }
          }
          frame "Launch Sequence Editor" {
            # "Launches the Sequence Editor for the specified TestStand version optionally with the specified environment."
            n140 = Variant To Data(error in=w333, type=T7 {"ITSDiscovery.lvclass"=refnum, "IProcess Executor.lvclass"=refnum, "Version"="", "Architecture"=enum."32bit", "Environment"=path "", "Wait Notifier"=refnum, "wait for reply"=FALSE} ("Launch Sequence Editor Argument"), Variant=w330) -> (data=w328:T7, error out=w331:errorcluster)
            n141 = Unbundle By Name(w328) -> ("IProcess Executor.lvclass"=w320:refnum<class "IProcess Executor.lvclass">, "Environment"=w314:path, "ITSDiscovery.lvclass"=w319:refnum<class "ITSDiscovery.lvclass">, "Version"=w316:string, "Architecture"=w315:T8, "Wait Notifier"=w327:refnum<notifier>, "wait for reply"=w326:bool)
            n142 = call "Get TSInstall by Version.vi"("Architecture"=w315, "Version"=w316, "ITSDiscovery in"=w319) -> ("error out"=w318:errorcluster, "TSInstall Out"=w322:T18)  [unwired: 7 in]
            n143 = call "Build SeqEdit Execution Plan.vi"("error in"=w318, "Environment"=w314, "TSInstall"=w322) -> ("error out"=w317:errorcluster, "Execution Plan"=w321:T26)  [unwired: 7 in]
            n144 = call-dynamic "Run.vi"("error in"=w317, "Execution Plan"=w321, "IProcess Executor in"=w320) -> ("error out"=w313:errorcluster)  [unwired: 7 in, 1 out]
            n145 = Bundle By Name(cluster=T22 {"error"={"status"=FALSE, "code"=0, "source"=""}, "Version"="", "Architecture"=enum."32bit", "Environment"=path ""} ("Launch Sequence Editor (Reply Payload)"), "Version"=w316, "Architecture"=w315, "Environment"=w314, "error"=w313) -> (w325:T22)
            n146 = Merge Errors(w331, w313) -> (w323:errorcluster)
            n147 = call "Launched SeqEdit.vi"("error in"=w313, "Reply Payload"=w325) -> ()  [unwired: 9 in, 1 out]
            n148 = case "DQMH_FIRE_NOTIFIER" shown="True" w326 {
              tunnel: w327 -> [_ w335]
              tunnel: w325 -> [_ w334]
              frame False {
              }
              frame True {
                n149 = Send Notification(notification=w334, notifier=w335) -> ()  [unwired: 1 in, 2 out]
              }
            }
          }
          frame "Delete Profile" {
            # "This request deletes the specified profile from the current profiles file."
            n150 = Variant To Data(error in=w349, type=T13 {"Name"="", "Wait Notifier"=refnum, "wait for reply"=FALSE} ("Delete Profile Argument"), Variant=w347) -> (data=w345:T13, error out=w348:errorcluster)
            n151 = Unbundle By Name(w345) -> ("Name"=w337:string, "Wait Notifier"=w344:refnum<notifier>, "wait for reply"=w343:bool)
            n152 = Unbundle By Name(w339) -> ("Profile File"=w338:path)
            n153 = call "Delete Profile from File.vi"("Name"=w337, "Profile File"=w338) -> ("error out"=w336:errorcluster)  [unwired: 9 in]
            n154 = Bundle By Name(cluster=T23 {"error"={"status"=FALSE, "code"=0, "source"=""}} ("Delete Profile (Reply Payload)"), "error"=w336) -> (w342:T23)
            n155 = Merge Errors(w348, w336) -> (w340:errorcluster)
            n156 = case "DQMH_FIRE_NOTIFIER" shown="True" w343 {
              tunnel: w344 -> [_ w351]
              tunnel: w342 -> [_ w350]
              frame False {
              }
              frame True {
                n157 = Send Notification(notification=w350, notifier=w351) -> ()  [unwired: 1 in, 2 out]
              }
            }
          }
          frame "Set Profiles File" {
            # "Error intentionally not broadcasted"
            # "This request was turned into a\nRequest and Wait for Reply to avoid\ntiming issues (DQMH module closed\nbefore INI-File actually written)"
            # "This request sets the specified profiles file in the cache INI file."
            n158 = Variant To Data(error in=w372, type=T14 {"File Path"=path "", "Wait Notifier"=refnum, "wait for reply"=FALSE} ("Set Profiles File Argument"), Variant=w370) -> (data=w368:T14, error out=w371:errorcluster)
            n159 = Unbundle By Name(w368) -> ("File Path"=w353:path, "Wait Notifier"=w367:refnum<notifier>, "wait for reply"=w366:bool)
            n160 = call "Cache INI File--constant.vi"() -> ("Cache INI File"=w362:path)  [unwired: 11 in]
            n161 = call <vilib>:"Open Config Data.vi"("configuration file path"=w362) -> ("error out"=w361:errorcluster, "refnum"=w360:T25)  [unwired: 8 in, 1 out]
            n162 = call "Cache INI Section--constant.vi"() -> ("Cache INI Section"=w359:string)  [unwired: 11 in]
            n163 = call "Profiles File Key--constant.vi"() -> ("Profiles File Key"=w358:string)  [unwired: 11 in]
            n164 = call-poly <vilib>:"Write Key.vi"("section"=w359, "error in (no error)"=w361, "value"=w353, "key"=w358, "refnum"=w360) -> ("error out"=w357:errorcluster, "refnum out"=w356:T25)  [unwired: 4 in, 1 out]
            n165 = call <vilib>:"Close Config Data.vi"("error in (no error)"=w357, "refnum"=w356) -> ("error out"=w352:errorcluster)  [unwired: 8 in, 1 out]
            n166 = Bundle By Name(cluster=w354, "Profile File"=w353) -> (w355:T2)
            n167 = Bundle By Name(cluster=T24 {"error"={"status"=FALSE, "code"=0, "source"=""}} ("Set Profiles File (Reply Payload)"), "error"=w352) -> (w365:T24)
            n168 = Merge Errors(w371) -> (w363:errorcluster)
            n169 = case "DQMH_FIRE_NOTIFIER" shown="True" w366 {
              tunnel: w367 -> [_ w374]
              tunnel: w365 -> [_ w373]
              frame False {
              }
              frame True {
                n170 = Send Notification(notification=w373, notifier=w374) -> ()  [unwired: 1 in, 2 out]
              }
            }
          }
          frame "---Copy This Frame---" {
            # "Duplicate this frame when creating new messages.  Change this comment in the duplicated frame to describe this message."
            n171 = Merge Errors(w377) -> (w376:errorcluster)
          }
          frame "---Exit and Error Handling---" {
            # "Separator - The following cases handle errors and exit messages."
          }
          frame "Simulate MHL Error" {
            # "#DQMH_HowTo The 'Simulate MHL Error' button  illustrates how the MHL handles errors. This event is instructional in nature and can be removed."
            # "Simulate an error occurring at the MHL"
            n172 = call "Module Name--constant.vi"() -> ("Module Name"=w381:string)  [unwired: 11 in]
            n173 = Format Into String(format string="Simulated error originating at Message Handling Loop in %s", w381) -> (resulting string=w382:string)  [unwired: 2 in, 1 out]
            n174 = call <vilib>:"Error Cluster From Error Code.vi"("show call chain? (False)"=TRUE, "error message (\"\")"=w382, "error code (0)"=5001) -> ("error out"=w386:errorcluster)  [unwired: 6 in]
            n175 = Merge Errors(w388, w386) -> (w387:errorcluster)
          }
          frame "Error" {
            # "#DQMH_CodeRecommended - If the module is running in standalone mode (External Launch = FALSE), this code will pop up an error dialog and call the 'Exit' message if an error occurs. Add more fine-grained error management here."
            # "Error - Check the error message data and respond accordingly. This message is sent by the \"Error Handler\" VIs at the end of each loop in this application."
            n176 = property on="Property Node" class="Module Admin"(reference=w391) -> ("Accessors:External Launch"=w390:bool)  [unwired: 1 in, 2 out]
            n177 = Variant To Data(error in=w399, type=errorcluster {"status"=FALSE, "code"=0, "source"=""} ("error constant"), Variant=w393) -> (data=w389:errorcluster, error out=w397:errorcluster)
            n178 = local write "error out"(w389) -> ()
            n179 = call "Error Reported.vi"("Error"=w389) -> ()  [unwired: 10 in, 1 out]
            n180 = case shown="True" w390 {
              tunnel: [w404 _] -> w396
              tunnel: w392 -> [w402 _]
              tunnel: w389 -> [w403 _]
              frame False {
                n181 = disable-structure shown="Default" {
                  disable-tunnel: w403 -> [w405 _]
                  frame condition #0 (active) {
                    # "If the module is running standalone, then pop up an error dialog and call the \"Exit\" message."
                    n182 = call <vilib>:"Simple Error Handler.vi"("error in (no error)"=w405) -> ()  [unwired: 4 in, 5 out]
                  }
                  frame condition #1 {
                    # "To prevent the Simple Error Handler VI from being loaded (e.g. when deploying to a Real-Time target), add the Conditional Disable Symbol \"DQMH_Disable_SEH\" to your project and set it to TRUE."
                  }
                }
                n183 = call-poly <vilib>:"Delacor_lib_QMH_Enqueue Message (poly).vi"("Priority Message? (F)"=TRUE, "Message"="Exit", "Message Queue in"=w402) -> ("error out"=w404:errorcluster)  [unwired: 7 in, 1 out]
              }
              frame True {
                # "If the module was launched externally, calling the Error Reported broadcast VI is the only action performed by the \"Error\" message. The module's caller can then process the error appropriately."
              }
            }
            n184 = Merge Errors(w397, w396) -> (w395:errorcluster)
          }
          frame "Exit" {
            w410 = 91  # 91: not all Exit messages will have an argument
            w412 = TRUE  # Stop the VI
            # "Release the message queue reference"
            # "#DQMH_CodeNeeded - Add any required cleanup code here."
            # "Exit - Exit the application."
            n185 = Variant To Data(error in=w420, type=T4 {"Origin"="", "Exit via Stop Module Req?"=FALSE, "Wait for Module to stop?"=FALSE} ("Stop Argument"), Variant=w411) -> (data=w408:T4, error out=w417:errorcluster)
            n186 = call <vilib>:"Clear Errors.vi"("error in (no error)"=w417, "specific error code to clear (0: all)"=w410) -> ("error out"=w419:errorcluster)  [unwired: 4 in, 1 out]
            n187 = control-ref of="This VI"() -> (w407:refnum<vi>)
            n188 = call-dynamic "Delacor_lib_QMH_Release Message Queue.vi"("error in"=w419, "Message Queue"=w414) -> ("error out"=w418:errorcluster)  [unwired: 9 in]
            n189 = call "Handle Exit.vi"("Stop Argument"=w408, "Admin in"=w406, "VI reference"=w407) -> ("error out"=w416:errorcluster)  [unwired: 7 in, 1 out]
            n190 = Merge Errors(w418, w416) -> (w415:errorcluster)
            n191 = call "Error Reported.vi"("Error"=w415) -> ()  [unwired: 10 in, 1 out]
          }
          frame Default {
            # "'Default' case only runs if there is a message that isn't defined in any of the other cases.  Output a programming error."
            n192 = call "Module Name--constant.vi"() -> ("Module Name"=w425:string)  [unwired: 11 in]
            n193 = Format Into String(format string="The invalid message string \"%s\" was received in the Message Handling Loop for module \"%s\".", w426, w425) -> (resulting string=w421:string)  [unwired: 2 in, 1 out]
            n194 = call <vilib>:"Error Cluster From Error Code.vi"("show call chain? (False)"=TRUE, "error message (\"\")"=w421, "error code (0)"=1) -> ("error out"=w428:errorcluster)  [unwired: 6 in]
            n195 = Merge Errors(w429, w428) -> (w430:errorcluster)
          }
        }
        n196 = call-dynamic "Delacor_lib_QMH_Error Handler - Message Handling Loop.vi"("error in"=w151, "Message Queue in"=w150) -> ("dup error in"=w152:errorcluster)  [unwired: 8 in, 1 out]
      }
    }
    frame Error {
      # "Synchronize Caller Events.vi will inform Start Module.vi that the module has launched and will let the code calling Start Module.vi register for broadcasts and would permit the caller receive the broadcast that an error occurred at launch time."
      n197 = call-dynamic "Delacor_lib_QMH_Release Message Queue.vi"("error in"=w438, "Message Queue"=w431) -> ("error out"=w437:errorcluster)  [unwired: 9 in]
      n198 = call "Synchronize Caller Events.vi"("Singleton Module Admin in"=w432) -> ("error out"=w439:errorcluster)  [unwired: 9 in, 1 out]
      n199 = call "Module Name--constant.vi"() -> ("Module Name"=w435:string)  [unwired: 11 in]
      n200 = Format Into String(format string="An error occurred during initialization. %s is no longer running.", w435) -> (resulting string=w433:string)  [unwired: 2 in, 1 out]
      n201 = Merge Errors(w437, w439) -> (w440:errorcluster)
      n202 = call "Error Reported.vi"("Additional Information"=w433, "Error"=w440) -> ()  [unwired: 9 in, 1 out]
    }
  }
  n203 = Merge Errors(w14, w17) -> (w13:errorcluster)
  n204 = call "Close Module.vi"("error in"=w13, "Module Admin in"=w8) -> ("error out"=w15:errorcluster, "External Launch"=w1:bool, "Module Admin out"=w2:refnum<class "Delacor_lib_QMH_Module Admin.lvclass">)  [unwired: 7 in]
  n205 = Unregister For Events(event registration refnum=w7, error in=w15) -> (error out=w12:errorcluster)
  "error out" <- w12
  n206 = case "External Launch?" shown="True" w1 {
    tunnel: w12 -> [_ w441]
    frame False {
    }
    frame True {
      n207 = case shown="No Error" w441 {
        frame No Error {
          n208 = invoke on="Invoke Node" class="VI" method="FP.Close"() -> ()  [unwired: 3 in, 3 out]
        }
        frame Error {
          n209 = disable-structure shown="Default" {
            frame condition #0 (active) {
              n210 = invoke class="VI" method="FP.Open"("Activate"=TRUE ("Activate?")) -> ()  [unwired: 4 in, 5 out]
            }
            frame condition #1 {
              # "Don't show panel on error if running inside a built EXE."
            }
          }
        }
      }
    }
  }
  n211 = local write "Module Admin"(w2) -> ()
